vi "checksum.vi"(8 "error in (no error)":errorcluster caption="Fehler (Eingang, kein Fehler)", 11 "Eingabe":string="NU,180;") -> (0 "Error Out":errorcluster caption="Fehler (Ausgang)", 3 "Ausgabe":string)   [LabVIEW 2013]
uses:
  EMV/res/dll/libchecksum.dll
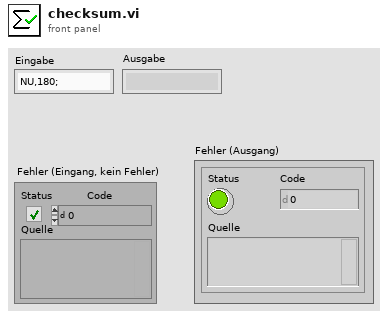
[diagram p1: front panel]
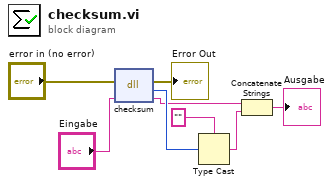
[diagram p0: block diagram]
diagram:
  n1 = dll-call lib="H:/sze/Bachelor Thesis/resourcen/Hauptprojekt/EMV/res/dll/libchecksum.dll" fn="checksum"(error in="error in (no error)", "befehl"="Eingabe") -> (error out=→"Error Out":errorcluster, "checksum"=w6:u8, "befehl"=w5:string)  [unwired: 2 in, 1 out]
  n2 = Type Cast(type="", x=w6) -> (*(type *) &x=w4:string)
  n3 = Concatenate Strings(w5, w4) -> (→"Ausgabe":string)
